vi "Core Action.vi"(8 "error in (no error)":errorcluster, 10 "SECS-II Class":refnum<class "SECS-II Class.lvclass">, 11 "10-On-Line Identification in":refnum<class "10-On-Line Identification.lvclass">) -> (0 "error out":errorcluster, 2 "SECS-II Class Out":refnum<class "SECS-II Class.lvclass">, 3 "10-On-Line Identification out":refnum<class "10-On-Line Identification.lvclass">)   [LabVIEW 2020, in "SECS Scenarios.lvlib" / "10-On-Line Identification.lvclass"]
uses:
  10-On-Line Identification.lvclass
  D:/Dropbox/SECS/SECS_GEM v1.1.0/Com/SECS Scenarios/Scenarios Class/Scenarios Class.lvclass
  SECS Communication/SECS-II Class/SECS-II Class.lvclass
  SECS Communication/S1 Message Class/S1 Message Class.lvclass
  D:/Dropbox/SECS/SECS_GEM v1.1.0/Com/SECS Communication/SECS-II Class/SECS-II Class.lvclass
  SECS Communication/S1 Message Class/S1F2.ctl
  Scenarios Class/Reply State.ctl
  Scenarios Class/Scenarios Class.lvclass/Scenarios Class.ctl
  Scenarios Class/Write Reply State.vi
  Scenarios Class/Read HSMS Class.vi
  SECS Communication/SECS Data Class/Get ECID Data.vi
  SECS Communication/SECS-II Class/Variant To Data_ASCII.vi
  SECS Communication/HSMS Class/HSMS Class.lvclass
  SECS Communication/SECS Data Class/SECS Data Class.lvclass
  Scenarios Class/Scenarios Class.lvclass
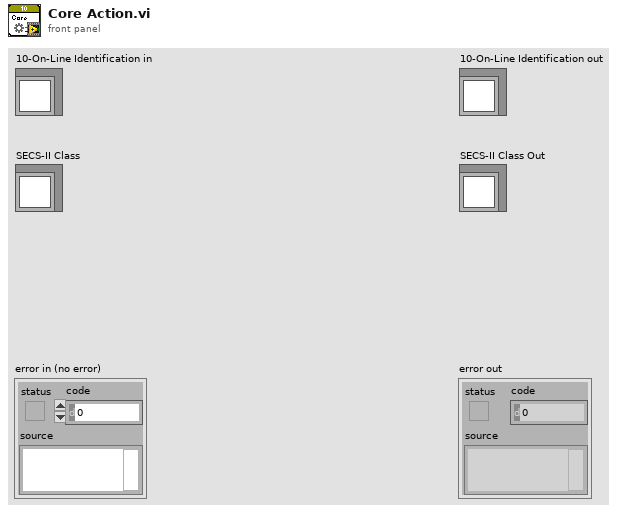
[diagram p1: front panel]
types:
  T1 = typedef "SECS Communication.lvlib/S1 Message Class.lvclass/S1F2.ctl" = cluster{"MDLN":string, "SOFTREV":string}
  T2 = typedef "SECS Communication.lvlib/SECS Data Class.lvclass/ECID Data.ctl" = cluster{"ECID":u32, "Name":string, "Description":string, "Format Code":T3, "Unit":string, "Max":dbl, "Min":dbl, "Default":string, "Source":string, "Data":variant}
  T3 = typedef "SECS Communication.lvlib/SECS-II Class.lvclass/Format Code.ctl" = enum16{"L", "A", "B", "Boolean", "J", "I1", "I2", "I4", "I8", "U1", "U2", "U4", "U8", "F4", "F8", "Char"}
  T4 = typedef "SECS Scenarios.lvlib/Scenarios Class.lvclass/Reply State.ctl" = enum16{"OK", "Illegal Data", "Unknown Stream", "Unknown Function", "Off-Line", "T3 Timeout", "Inner-Timeout"}
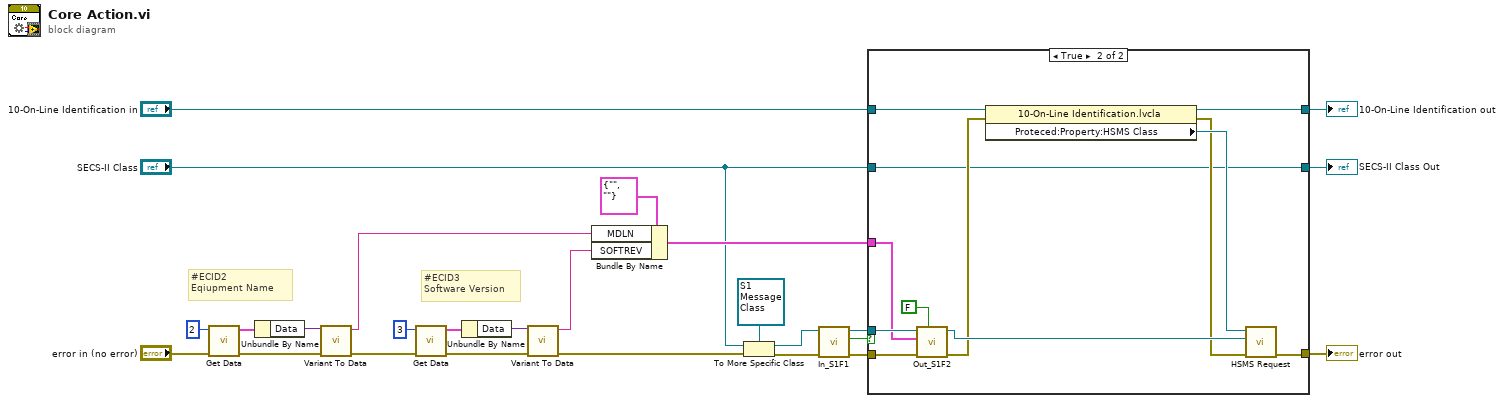
[diagram p0: block diagram]
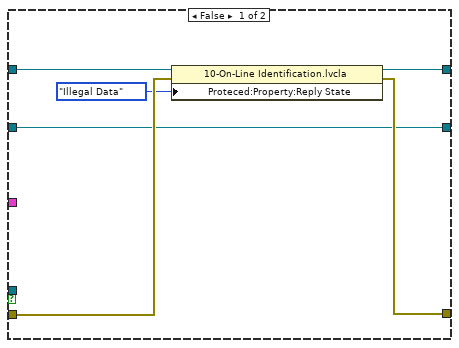
[diagram p2: hidden frame]
diagram:
  # "#ECID3\nSoftware Version"
  # "#ECID2\nEqiupment Name"
  n1 = call-poly "Get Data.vi"("error in"="error in (no error)", "ECID"=u32 2) -> ("error out"=w24:errorcluster, "ECID Data"=w25:T2)  [unwired: 7 in, 1 out]
  n2 = Unbundle By Name(w25) -> ("Data"=w23:variant)
  n3 = call-poly "Variant To Data.vi"("error in (no error)"=w24, "Variant"=w23) -> ("error out"=w17:errorcluster, "Data"=w16:string)  [unwired: 7 in, 1 out]
  n4 = call-poly "Get Data.vi"("error in"=w17, "ECID"=u32 3) -> ("error out"=w19:errorcluster, "ECID Data"=w18:T2)  [unwired: 7 in, 1 out]
  n5 = Unbundle By Name(w18) -> ("Data"=w20:variant)
  n6 = call-poly "Variant To Data.vi"("error in (no error)"=w19, "Variant"=w20) -> ("error out"=w1:errorcluster, "Data"=w15:string)  [unwired: 7 in, 1 out]
  n7 = Bundle By Name(cluster=T1 {"MDLN"="", "SOFTREV"=""} ("S1F2"), "MDLN"=w16, "SOFTREV"=w15) -> (w8:T1)
  n8 = To More Specific Class(target class=refnum<class "S1 Message Class.lvclass"> refnum ("S1 Message Class in"), reference="SECS-II Class", error in=w1) -> (specific class reference=w12:refnum<class "S1 Message Class.lvclass">, error out=w13:errorcluster)
  n9 = call "In_S1F1.vi"("error in (no error)"=w13, "S1 Message Class in"=w12) -> ("error out"=w10:errorcluster, "OK?"=w7:bool, "S1 Message Class out"=w9:refnum<class "S1 Message Class.lvclass">)  [unwired: 7 in]
  n10 = case shown="True" w7 {
    tunnel: w10 -> [w30 w44]
    tunnel: w9 -> [_ w43]
    tunnel: w8 -> [_ w42]
    tunnel: [w29 w39] -> w5
    tunnel: "10-On-Line Identification in" -> [w32 w38]
    tunnel: [w31 w37] -> w6
    tunnel: "SECS-II Class" -> [w27 w33]
    tunnel: [w27 w33] -> w2
    frame False {
      n11 = property class="10-On-Line Identification.lvcla"(reference=w32, error in=w30, "Proteced:Property:Reply State"=Reply_State."Illegal Data" ("Reply State")) -> (reference out=w31:refnum<class "10-On-Line Identification.lvclass">, error out=w29:errorcluster)
    }
    frame True {
      n12 = call "Out_S1F2.vi"("Host"=FALSE, "error in (no error)"=w44, "S1F2"=w42, "S1 Message Class in"=w43) -> ("error out"=w36:errorcluster, "S1 Message Class out"=w41:refnum<class "S1 Message Class.lvclass">)  [unwired: 6 in]
      n13 = property class="10-On-Line Identification.lvcla"(reference=w38, error in=w36) -> (reference out=w37:refnum<class "10-On-Line Identification.lvclass">, error out=w34:errorcluster, "Proteced:Property:HSMS Class"=w35:refnum<class "HSMS Class.lvclass">)
      n14 = call "HSMS Request.vi"("error in (no error)"=w34, "SECS-II Class In"=w41, "HSMS Class in"=w35) -> ("error out"=w39:errorcluster)  [unwired: 7 in, 1 out]
    }
  }
  "error out" <- w5
  "10-On-Line Identification out" <- w6
  "SECS-II Class Out" <- w2
